vi "MessageDestination.vi"(11 "Robot":T1={"id"=0, "function"=enum."Attacker", "x"=0.0, "y"=0.0, "orientation"=0.0, "v_tangent"=0.0, "v_normal"=0.0, "v_ang"=0.0, "kick_x"=0.0, "kick_z"=0.0, "dribble"=FALSE, "Timestamp"=timestamp(0 s since 1904-01-01), "estimatives"={"est_v_tangent"=0.0, "est_v_normal"=0.0, "est_vx"=0.0, "est_vy"=0.0, "Pos Robot Est"=[]}, "dest_x_kick"=0.0, "dest_y_kick"=0.0, "Gap Coord"=[], "States"=enum."GoToTangent", "Path "=[], "Path  Smooth"=[], "Dest"=[], "vx_desired"=0.0, "vy_desired"=0.0, "slowBehavior"=FALSE, "VSSStates"=enum."Pass"}) -> (1 "Array":u8[](array[numeric]))   [LabVIEW 2020]
uses:
  Vision_class/Old vision/Controls/AI Robot.ctl
  Vision_class/Old vision/Controls/Functions Enum.ctl
  Vision_class/Old vision/Controls/AttackerStates.ctl
  Vision_class/Old vision/Controls/PathDests.ctl
  Vision_class/Old vision/Controls/PathDest.ctl
  Game_class/Navigation/VSSNavigation/VSSAttackerStates.ctl
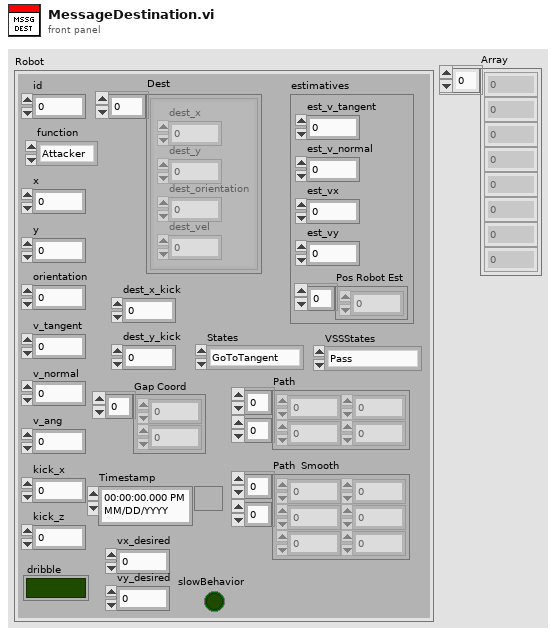
[diagram p1: front panel]
types:
  T1 = typedef "AI Robot.ctl" = cluster{"id":u32, "function":T2, "x":dbl, "y":dbl, "orientation":dbl, "v_tangent":dbl, "v_normal":dbl, "v_ang":dbl, "kick_x":dbl, "kick_z":dbl, "dribble":bool, "Timestamp":timestamp, "estimatives":cluster{"est_v_tangent":dbl, "est_v_normal":dbl, "est_vx":dbl, "est_vy":dbl, "Pos Robot Est":dbl[]}, "dest_x_kick":dbl, "dest_y_kick":dbl, "Gap Coord":dbl[], "States":T3, "Path ":dbl[][], "Path  Smooth":dbl[][], "Dest":T4, "vx_desired":dbl, "vy_desired":dbl, "slowBehavior":bool, "VSSStates":T6}
  T2 = typedef "Functions Enum.ctl" = enum16{"2nd Striker", "Attacker", "Goalie", "Defender", "Striker", "Goto 0", "Dummy", "Kicker", "ZigZag 0", "ZigZag 1", "ZigZag 2", "ZigZag 3", "ZigZag 4", "ZigZag 5", "ZigZag 6", "ZigZag 7", "ZigZag 8", ""}
  T3 = typedef "AttackerStates.ctl" = enum16{"Pass", "GoToTangent", "BallGetting", "GoToKick", ""}
  T4 = typedef "PathDests.ctl" = T5[]
  T5 = typedef "PathDest.ctl" = cluster{"dest_x":dbl, "dest_y":dbl, "dest_orientation":dbl, "dest_vel":dbl}
  T6 = typedef "VSSAttackerStates.ctl" = enum16{"Pass", "GoToTangent", "BallGetting", "GoToKick", "Rotate anti-clockwise", "Rotate Clockwise", ""}
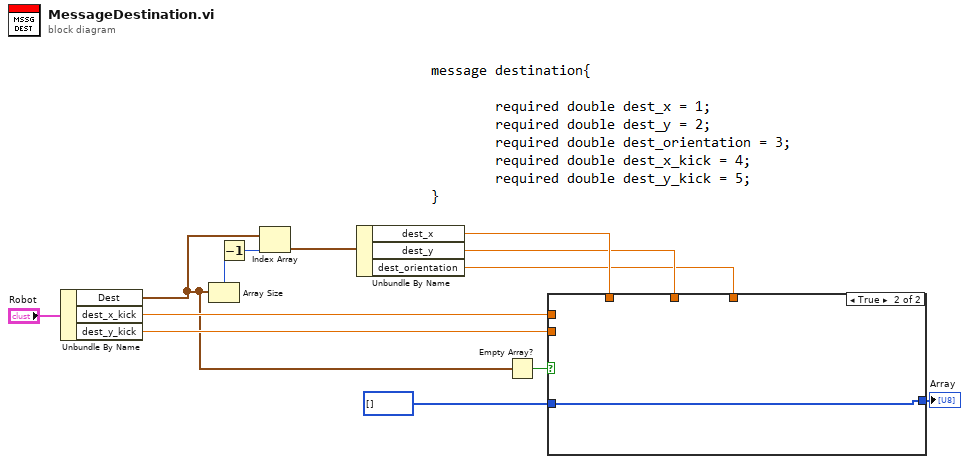
[diagram p0: block diagram]
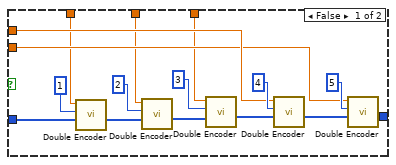
[diagram p2: hidden frame]
diagram:
  n1 = Unbundle By Name("Robot") -> ("Dest"=w1:T4, "dest_x_kick"=w11:dbl, "dest_y_kick"=w10:dbl)
  n2 = Array Size(array=w1) -> (size(s)=w7:i32)
  n3 = Decrement(x=w7) -> (x-1=w8:i32)
  n4 = Index Array(array=w1, index=w8) -> (element=w2:T5)
  n5 = Unbundle By Name(w2) -> ("dest_x"=w6:dbl, "dest_y"=w5:dbl, "dest_orientation"=w4:dbl)
  n6 = Empty Array?(array=w1) -> (empty?=w3:bool)
  n7 = case shown="True" w3 {
    tunnel: u8[] [] ("Array In") -> [w29 w30]
    tunnel: w11 -> [w20 _]
    tunnel: w10 -> [w19 _]
    tunnel: [w18 w30] -> w9
    tunnel: w6 -> [w17 _]
    tunnel: w5 -> [w15 _]
    tunnel: w4 -> [w14 _]
    frame False {
      n8 = call "Double Encoder.vi"("Array In"=w29, "Key"=u32 1, "Value"=w17) -> ("Array"=w27:u8[])  [unwired: 8 in]
      n9 = call "Double Encoder.vi"("Array In"=w27, "Key"=u32 2, "Value"=w15) -> ("Array"=w25:u8[])  [unwired: 8 in]
      n10 = call "Double Encoder.vi"("Array In"=w25, "Key"=u32 3, "Value"=w14) -> ("Array"=w23:u8[])  [unwired: 8 in]
      n11 = call "Double Encoder.vi"("Array In"=w23, "Key"=u32 4, "Value"=w20) -> ("Array"=w21:u8[])  [unwired: 8 in]
      n12 = call "Double Encoder.vi"("Array In"=w21, "Key"=u32 5, "Value"=w19) -> ("Array"=w18:u8[])  [unwired: 8 in]
    }
    frame True {
    }
  }
  "Array" <- w9
